vi "Translator.File.MatchStrings (Array).vi"(4 "sort? (T)":bool=TRUE, 5 "progressbar":refnum<vi>, 7 "group":string, 8 "error in":errorcluster, 9 "labels":string[](array[string]), 10 "default values":string[](array[string]), 11 "refnum in":T1) -> (0 "error out":errorcluster, 1 "#added":i32, 2 "values out":string[](array[string]), 3 "refnum out":T1)   [LabVIEW 2019, in "Tools.lvlib"]
uses:
  Tools.lvlib
  <vilib>/Utility/config.llb/Config Data RefNum.ctl
  <vilib>/Utility/config.llb/Read Key (String).vi
  <vilib>/Utility/config.llb/Write Key (String).vi
  <vilib>/Utility/config.llb/NI_LVConfig.lvlib
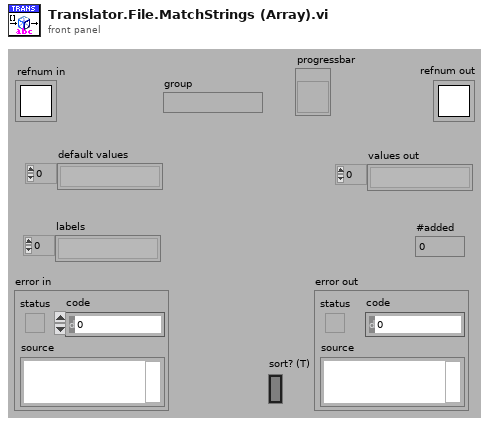
[diagram p1: front panel]
types:
  T1 = typedef "NI_LVConfig.lvlib/Config Data RefNum.ctl" = refnum<k1>
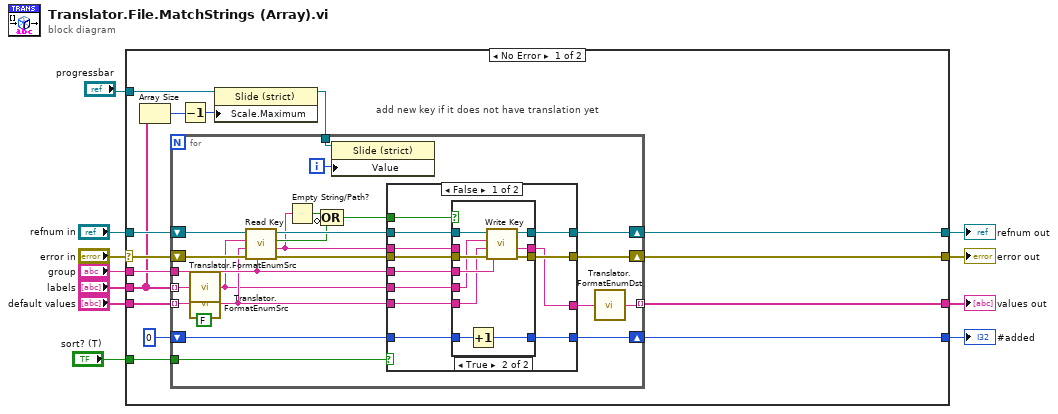
[diagram p0: block diagram]
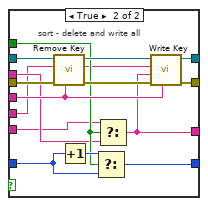
[diagram p3: hidden frame]
diagram:
  n1 = case shown="No Error" "error in" {
    selector: "error in" -> [w21 w91]
    tunnel: "refnum in" -> [w20 w92]
    tunnel: [w25 _] -> w10
    tunnel: [w13 w92] -> w9
    tunnel: [w12 w91] -> w8
    tunnel: [w24 w90] -> w7
    tunnel: "group" -> [w23 _]
    tunnel: "labels" -> [w17 _]
    tunnel: "default values" -> [w22 w90]
    tunnel: "progressbar" -> [w16 _]
    tunnel: "sort? (T)" -> [w14 _]
    frame No Error {
      # "add new key if it does not have translation yet"
      n2 = Array Size(array=w17) -> (size(s)=w19:i32)
      n3 = Decrement(x=w19) -> (x-1=w18:i32)
      n4 = property on="Property Node" class="Slide (strict)"(reference=w16, "Scale.Maximum"=w18) -> (reference out=w15:refnum<vi>)  [unwired: 1 in, 1 out]
      n5 = for {
        tunnel: w23 -> [w45]
        tunnel: w17 -> [w44] mode=indexing
        shift-right: [w27] -> w12
        shift-left: w21 -> [w49]
        shift-right: [w28] -> w13
        shift-left: w20 -> [w48]
        tunnel: [w30] -> w24 mode=indexing
        shift-right: [w36] -> w25
        shift-left: 0 -> [w37]
        tunnel: w22 -> [w43] mode=indexing
        tunnel: w15 -> [w34]
        tunnel: w14 -> [w31]
        i -> [w32]
        n6 = call "Translator.FormatEnumSrc.vi"("text in"=w44) -> ("text out"=w33:string)  [unwired: 1 in]
        n7 = call "Translator.FormatEnumSrc.vi"("text in"=w43, "quotas?(T)"=FALSE) -> ("text out"=w42:string)
        n8 = call-poly <vilib>:"Read Key.vi"("section"=w45, "error in (no error)"=w49, "default value"=w42, "key"=w33, "refnum"=w48) -> ("error out"=w47:errorcluster, "value"=w38:string, "found?"=w39:bool, "refnum out"=w46:T1)  [unwired: 3 in]
        n9 = Empty String/Path?(string/path=w38) -> (empty?=w41:bool)
        n10 = Compound Arithmetic op=OR(w41, invert w39) -> (w40:bool)
        n11 = property on="Property Node" class="Slide (strict)"(reference=w34, "Value"=w32) -> ()  [unwired: 1 in, 2 out]
        n12 = case shown="False" w31 {
          tunnel: w47 -> [w61 w89]
          tunnel: [w60 w84] -> w27
          tunnel: w46 -> [w59 w88]
          tunnel: [w58 w86] -> w28
          tunnel: w45 -> [w57 w83]
          tunnel: w42 -> [w56 w77]
          tunnel: w40 -> [w55 w79]
          tunnel: w38 -> [w54 w78]
          tunnel: w37 -> [w53 w82]
          tunnel: [w52 w80] -> w36
          tunnel: w33 -> [w51 w75]
          tunnel: [w50 w76] -> w29
          frame False {
            n13 = case shown="True" w55 {
              tunnel: w61 -> [w64 w74]
              tunnel: [w64 w73] -> w60
              tunnel: w59 -> [w65 w72]
              tunnel: [w65 w71] -> w58
              tunnel: w57 -> [_ w70]
              tunnel: w56 -> [_ w66]
              tunnel: w54 -> [w63 _]
              tunnel: w51 -> [_ w69]
              tunnel: [w63 w66] -> w50
              tunnel: w53 -> [w62 w68]
              tunnel: [w62 w67] -> w52
              frame False {
              }
              frame True {
                n14 = Increment(x=w68) -> (x+1=w67:i32)
                n15 = call-poly <vilib>:"Write Key.vi"("section"=w70, "error in (no error)"=w74, "value"=w66, "key"=w69, "refnum"=w72) -> ("error out"=w73:errorcluster, "refnum out"=w71:T1)  [unwired: 4 in, 1 out]
              }
            }
          }
          frame True {
            # "sort - delete and write all"
            n16 = call <vilib>:"Remove Key.vi"("section"=w83, "error in (no error)"=w89, "key"=w75, "refnum"=w88) -> ("error out"=w85:errorcluster, "refnum out"=w87:T1)  [unwired: 5 in, 1 out]
            n17 = Increment(x=w82) -> (x+1=w81:i32)
            n18 = Select(t=w81, s=w79, f=w82) -> (s? t:f=w80:i32)
            n19 = Select(t=w77, s=w79, f=w78) -> (s? t:f=w76:string)
            n20 = call-poly <vilib>:"Write Key.vi"("section"=w83, "error in (no error)"=w85, "value"=w76, "key"=w75, "refnum"=w87) -> ("error out"=w84:errorcluster, "refnum out"=w86:T1)  [unwired: 4 in, 1 out]
          }
        }
        n21 = call "Translator.FormatEnumDst.vi"("text in"=w29) -> ("text out"=w30:string)
      }
    }
    frame Error {
    }
  }
  "#added" <- w10
  "refnum out" <- w9
  "error out" <- w8
  "values out" <- w7
